vi "ENPH354_A4Q2.vi"() -> ()   [LabVIEW 2020]
uses:
  <vilib>/Analysis/baseanly.llb/Mean (DBL).vi
  <vilib>/Utility/file.llb/Read Delimited Spreadsheet (DBL).vi
  <vilib>/Analysis/NI_AALBase.lvlib
panel:
  in  "Save Corrected Data":path
  out "Corrected Data\nWLED Emission Spec":cluster{dbl[], dbl[]}(graph)
  out "Corrected Data Array":dbl[][](array[numeric])
  out "Avg Count":dbl
  out "Original Data Array":dbl[][](array[numeric])
  in  "WLED Emission Spec":path
  out "Original Data\nWLED Emission Spec":cluster{"X":dbl[], "Y":dbl[]}[](graph)
  # "ENPH354 Assignment 4 Q2"
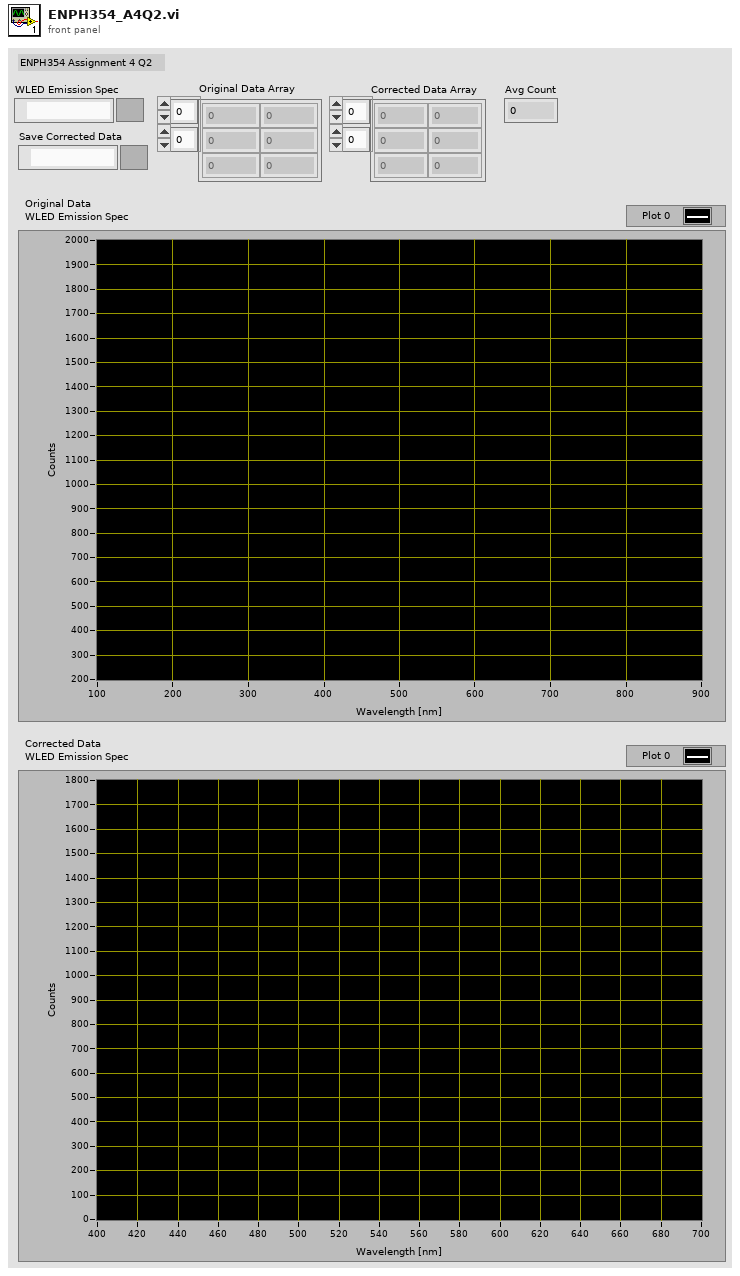
[diagram p1: front panel]
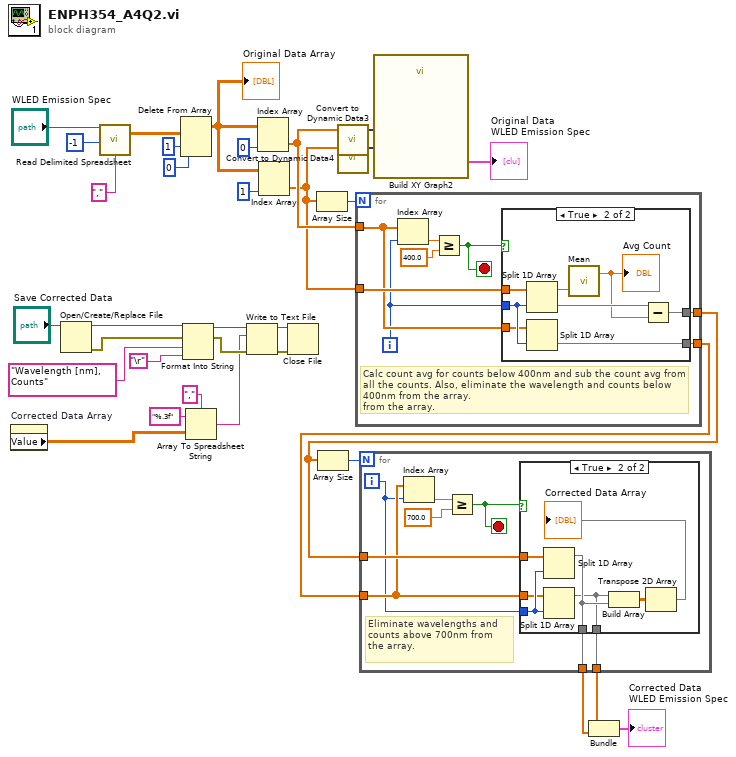
[diagram p0: block diagram]
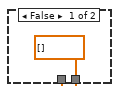
[diagram p2: hidden frame]
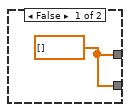
[diagram p3: hidden frame]
diagram:
  n1 = property on="Corrected Data Array" class="Arr (strict)"() -> ("Value"=w6:dbl[][])  [unwired: 2 in, 2 out]
  n2 = Open/Create/Replace File(file path (use dialog)="Save Corrected Data") -> (refnum out=w16:refnum<file>, error out=w13:errorcluster)  [unwired: 5 in, 1 out]
  n3 = call-poly <vilib>:"Read Delimited Spreadsheet.vi"("file path (dialog if empty)"="WLED Emission Spec", "number of rows (all:-1)"=-1, "delimiter (\\t)"="," ("delimiter (\\t)")) -> ("all rows"=w30:dbl[][])  [unwired: 7 in, 5 out]
  n4 = Delete From Array(array=w30, length=1, index (row)=0) -> (array with subset deleted=w22:dbl[][])  [unwired: 1 in, 1 out]
  "Original Data Array" <- w22
  n5 = Format Into String(initial string=w16, error in=w13, "Wavelength [nm], Counts", "\r") -> (resulting string=w15:refnum<file>, error out=w12:errorcluster)  [unwired: 1 in]
  n6 = Array To Spreadsheet String(delimiter (Tab)=",", array=w6, 3:"%.3f" ("format string")) -> (spreadsheet string=w8:string)
  n7 = Write to Text File(file (use dialog)=w15, text=w8, error in=w12) -> (refnum out=w14:refnum<file>, error out=w11:errorcluster)  [unwired: 1 in, 1 out]
  n8 = Index Array(array=w22, index (col)=0) -> (element=w23:dbl[])  [unwired: 1 in]
  n9 = Index Array(array=w22, index (col)=1) -> (element=w19:dbl[])  [unwired: 1 in]
  n10 = Close File(refnum=w14, error in=w11) -> ()  [unwired: 2 out]
  n11 = Array Size(array=w19) -> (size(s)=w21:i32)
  n12 = call "Convert to Dynamic Data3"("Array"=w23) -> ("Dynamic Data Type"=w25:dynamicdata)  [unwired: 3 in]
  n13 = call "Convert to Dynamic Data4"("Array"=w19) -> ("Dynamic Data Type"=w24:dynamicdata)  [unwired: 3 in]
  n14 = for {
    N: w21 -> [_]
    tunnel: w23 -> [w38]
    tunnel: w19 -> [w40]
    tunnel: [w37] -> w18
    tunnel: [w36] -> w17
    i -> [w35]
    stop <- w39 stop-if-true
    # "Calc count avg for counts below 400nm and sub the count avg from all the counts. Also, eliminate the wavelength and counts below 400nm from the array.\nfrom the array."
    n15 = Index Array(array=w38, index=w35) -> (element=w42:dbl)
    n16 = Greater Or Equal?(x=w42, y=400.0) -> (x >= y?=w39:bool)
    n17 = case shown="True" w39 {
      tunnel: w40 -> [_ w51]
      tunnel: w35 -> [_ w49]
      tunnel: w38 -> [_ w48]
      tunnel: [w43 w47] -> w37
      tunnel: [w43 w46] -> w36
      frame False {
        w43 = dbl[] []
      }
      frame True {
        n18 = Split 1D Array(array=w51, index=w49) -> (first subarray=w50:dbl[], second subarray=w45:dbl[])
        n19 = Split 1D Array(array=w48, index=w49) -> (second subarray=w47:dbl[])  [unwired: 1 out]
        n20 = call-poly <vilib>:"Mean.vi"("X"=w50) -> ("mean"=w44:dbl)  [unwired: 1 out]
        "Avg Count" <- w44
        n21 = Subtract(x=w45, y=w44) -> (x-y=w46:dbl[])
      }
    }
  }
  n22 = Array Size(array=w17) -> (size(s)=w20:i32)
  n23 = for {
    N: w20 -> [_]
    tunnel: w17 -> [w56]
    tunnel: w18 -> [w55]
    tunnel: [w53] -> w3
    tunnel: [w52] -> w4
    i -> [w54]
    stop <- w57 stop-if-true
    # "Eliminate wavelengths and \ncounts above 700nm from\nthe array."
    n24 = Index Array(array=w55, index=w54) -> (element=w59:dbl)
    n25 = Greater Or Equal?(x=w59, y=700.0) -> (x >= y?=w57:bool)
    n26 = case shown="True" w57 {
      tunnel: w56 -> [_ w67]
      tunnel: w55 -> [_ w65]
      tunnel: w54 -> [_ w66]
      tunnel: [w60 w62] -> w53
      tunnel: [w60 w61] -> w52
      frame False {
        w60 = dbl[] []
      }
      frame True {
        n27 = Split 1D Array(array=w67, index=w66) -> (first subarray=w62:dbl[])  [unwired: 1 out]
        n28 = Split 1D Array(array=w65, index=w66) -> (first subarray=w61:dbl[])  [unwired: 1 out]
        n29 = Build Array(w61, w62) -> (w63:dbl[][])
        n30 = Transpose 2D Array(2D array=w63) -> (transposed array=→"Corrected Data Array":dbl[][])
      }
    }
  }
  n31 = call "Build XY Graph2"("Y Input"=w24, "X Input"=w25) -> ("XY Graph"=→"Original Data\nWLED Emission Spec":cluster{"X":dbl[], "Y":dbl[]}[])  [unwired: 8 in, 1 out]
  n32 = Bundle(w4, w3) -> (→"Corrected Data\nWLED Emission Spec":cluster{dbl[], dbl[]})  [unwired: 1 in]
